vi "Year2018_Q2.vi"() -> ()   [LabVIEW 2015]
panel:
  in  "Setting":dbl
  out "Alarm":bool
  in  "Room C":bool
  in  "Room  B":bool
  in  "Room A":bool
  in  "stop":bool
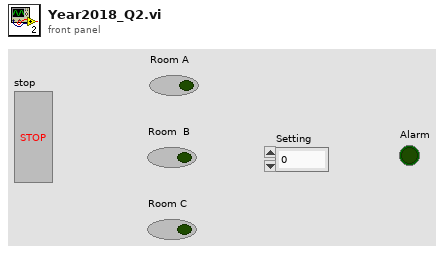
[diagram p1: front panel]
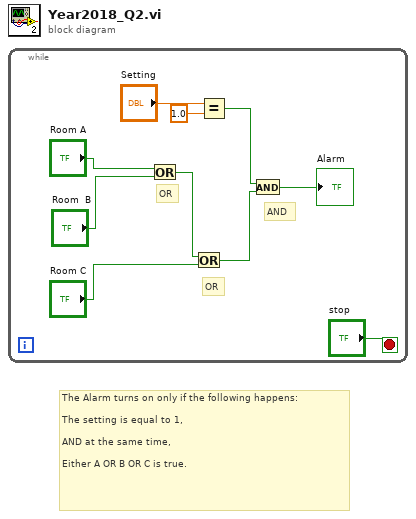
[diagram p0: block diagram]
diagram:
  # "The Alarm turns on only if the following happens:\n\nThe setting is equal to 1,\n\nAND at the same time,\n\nEither A OR B OR C is true."
  n1 = while {
    stop <- "stop" stop-if-true
    # "OR"
    # "OR"
    # "AND"
    n2 = Or(x="Room A", y="Room  B") -> (x .or. y?=w5:bool)
    n3 = Or(x=w5, y="Room C") -> (x .or. y?=w2:bool)
    n4 = Equal?(x="Setting", y=1.0) -> (x = y?=w3:bool)
    n5 = And(x=w3, y=w2) -> (x .and. y?=→"Alarm":bool)
  }
